vi "Facade.vi"(0 "Data In":T16={"Type"=enum."Tone", "Tone"={"Frequency (kHz)"=0.0, "Phase (cycles)"=0.0, "Random phase"=FALSE}, "Pulse Train"={"Pulse width (us)"=0.0, "Pulse rate (Hz)"=0.0, "Gap (ms)"=0.0, "Polarity"=enum."POS", "PT State"={"Template"=[], "Nperiod"=0, "Index"=0, "Pulse Rate (Hz)"=0.0, "Phase (cycles)"=0.0, "Noff"=0}, "Asynch"=FALSE}, "Noise"={"Properties"={"InvFilt"=FALSE, "Aweight"=FALSE, "Seed"=0, "Tokens"=0, "Brickwall"=FALSE}, "Data"={"TokenNum"=0}}, "File"={"Filename"=path "", "Signal"=[], "Channel"=0, "stream"=FALSE, "offset"=0, "nreps"=0, "loops"=0, "Randomize"=FALSE, "order"=[], "Seed"=0, "Tokens"=0}, "FMSweep"={"Rate (oct/s)"=0.0, "Fmin (Hz)"=0.0, "Fmax (Hz)"=0.0, "Ramp (ms)"=0.0, "Linear"=FALSE}, "Chirp Train"={"Params"={"Fmin (kHz)"=4.0, "Fmax (kHz)"=64.0, "Compensate"=FALSE, "Duration (ms)"=2.0}, "Data"={"WF"=[]}}, "Complex Tone"={"Params"={"F0 (Hz)"=0.0, "Band"={"Flow (Hz)"=0.0, "Fhigh (Hz)"=0.0}, "Phase"=enum."Cosine", "Min F0 (Hz)"=0.0, "Max F0 (Hz)"=0.0, "ContinRandPhase"=FALSE, "Max peak factor"=inf, "Max mod depth"=2.0, "MinHarmNum"=0, "MaxHarmNum"=0, "Level Mode"=enum."per component", "% jitter"=0.0}, "Data"={"Ncomp"=0, "MinHarm"=0, "Phase"=[], "Amplitude"=[], "Npts/frame"=0, "Last F0"=0.0, "Fmin"=0.0, "Fmax"=0.0, "Lslope"=0.0, "randphase"=FALSE, "overall rms"=FALSE, "fmult"=[], "jittered"=FALSE}}, "FM"={"Carrier (kHz)"=0.0, "ModRate (Hz)"=0.0, "Depth (Hz)"=0.0, "Phase (cycles)"=0.0}, "Vowel"={"Freqs"="", "Set level"=enum."Total", "Freq"=[], "weights"=[]}, "Ramp"={"Duration (ms)"=0.0}}, 2 "Display State In":T13, 3 "Container State":T15) -> (6 "Data Out":T16={"Type"=enum."Tone", "Tone"={"Frequency (kHz)"=0.0, "Phase (cycles)"=0.0, "Random phase"=FALSE}, "Pulse Train"={"Pulse width (us)"=0.0, "Pulse rate (Hz)"=0.0, "Gap (ms)"=0.0, "Polarity"=enum."POS", "PT State"={"Template"=[], "Nperiod"=0, "Index"=0, "Pulse Rate (Hz)"=0.0, "Phase (cycles)"=0.0, "Noff"=0}, "Asynch"=FALSE}, "Noise"={"Properties"={"InvFilt"=FALSE, "Aweight"=FALSE, "Seed"=0, "Tokens"=0, "Brickwall"=FALSE}, "Data"={"TokenNum"=0}}, "File"={"Filename"=path "", "Signal"=[], "Channel"=0, "stream"=FALSE, "offset"=0, "nreps"=0, "loops"=0, "Randomize"=FALSE, "order"=[], "Seed"=0, "Tokens"=0}, "FMSweep"={"Rate (oct/s)"=0.0, "Fmin (Hz)"=0.0, "Fmax (Hz)"=0.0, "Ramp (ms)"=0.0, "Linear"=FALSE}, "Chirp Train"={"Params"={"Fmin (kHz)"=4.0, "Fmax (kHz)"=64.0, "Compensate"=FALSE, "Duration (ms)"=2.0}, "Data"={"WF"=[]}}, "Complex Tone"={"Params"={"F0 (Hz)"=0.0, "Band"={"Flow (Hz)"=0.0, "Fhigh (Hz)"=0.0}, "Phase"=enum."Cosine", "Min F0 (Hz)"=0.0, "Max F0 (Hz)"=0.0, "ContinRandPhase"=FALSE, "Max peak factor"=inf, "Max mod depth"=2.0, "MinHarmNum"=0, "MaxHarmNum"=0, "Level Mode"=enum."per component", "% jitter"=0.0}, "Data"={"Ncomp"=0, "MinHarm"=0, "Phase"=[], "Amplitude"=[], "Npts/frame"=0, "Last F0"=0.0, "Fmin"=0.0, "Fmax"=0.0, "Lslope"=0.0, "randphase"=FALSE, "overall rms"=FALSE, "fmult"=[], "jittered"=FALSE}}, "FM"={"Carrier (kHz)"=0.0, "ModRate (Hz)"=0.0, "Depth (Hz)"=0.0, "Phase (cycles)"=0.0}, "Vowel"={"Freqs"="", "Set level"=enum."Total", "Freq"=[], "weights"=[]}, "Ramp"={"Duration (ms)"=0.0}}, 7 "Display State Out":T13, 8 "Action":T12)   [LabVIEW 2020, in "Waveform (G3).xctl"]
uses:
  Waveform (G3).xctl
  Waveform Data.ctl
  Waveform VIs/Waveform Enum (V3).ctl
  Tone (G3)/Tone.Properties.ctl
  Waveform VIs/Pulse Train VIs/Pulse Train Params.ctl
  Waveform VIs/Pulse Train VIs/Pulse Polarity.ctl
  Waveform VIs/Pulse Train VIs/PT-Continuous State.ctl
  Waveform VIs/Noise VIs/Noise (G3).ctl
  Waveform VIs/Noise VIs/Noise (G3).Properties.ctl
  Waveform VIs/Noise VIs/Noise (G3).Data.ctl
  Waveform VIs/File VIs/StimFile-Params.ctl
  Waveform VIs/FM Sweep VIs/FM Sweep Params.ctl
  Waveform VIs/Chirp Train VIs/Chirp Train.ctl
  Waveform VIs/Chirp Train VIs/Chirp Train Params.ctl
  Waveform VIs/Complex Tone VIs/CT-Params.ctl
  Waveform VIs/Complex Tone VIs/CT-Phase Enum.ctl
  Waveform VIs/Complex Tone VIs/CT-Runtime Data.ctl
  FM Tone/Data.ctl
  Vowel/Vowel.Properties.ctl
  Waveform VIs/Ramp VIs/Ramp.Properties.ctl
  <vilib>/_xctls/Container State.ctl
  State.ctl
  Utility VIs/Controls/KRing/KRing.xctl
  Tone (G3)/Tone (G3).xctl
  Noise (G3)/Noise (G3).xctl
  Noise (G3)/Noise (G3) - Persistent.ctl
  <vilib>/_xctls/Action.ctl
  FM Tone/FM Tone.xctl
  Vowel/Vowel.xctl
  <vilib>/_xctls/XControlSupport.lvlib
panel:
  out "display state signal":bool
  in  "Waveform":i16(xcontrol)
  in  "Tab Control":T1(tab)
  in  "Tone (G3)":T2(xcontrol)
  in  "Noise (G3)":T3(xcontrol)
  in  "Pulse Train Params":T4
  in  "File Params":T7
  in  "FMSweep":T8
  in  "Chirp Train Params":T9={"Fmin (kHz)"=4.0, "Fmax (kHz)"=64.0, "Compensate"=FALSE, "Duration (ms)"=2.0}
  in  "FM Tone":T10(xcontrol)
  in  "Vowel":T11(xcontrol)
  in  "Ramp":cluster{"Duration (ms)":dbl}
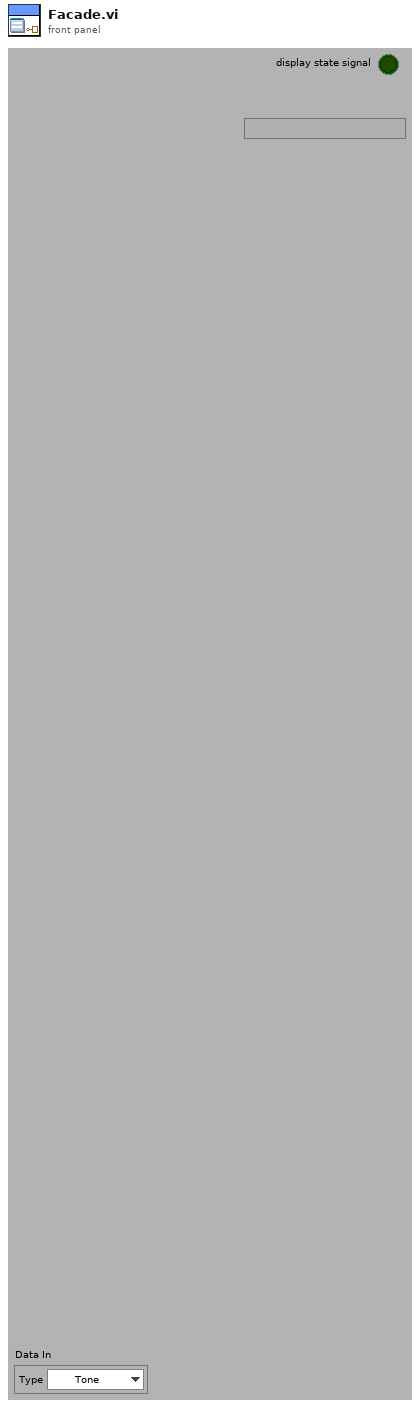
[diagram p1: front panel]
types:
  T1 = enum32{"OFF", "Tone", "Noise", "Pulse train", "File", "FM Sweep", "Chirp", "Complex Tone", "FM Tone", "Vowel", "Ramp"}
  T2 = cluster{"Frequency (kHz)":dbl, "Phase (cycles)":dbl, "Random phase":bool}
  T3 = cluster{"InvFilt":bool, "Aweight":bool, "Seed":i32, "Tokens":i32, "Brickwall":bool}
  T4 = typedef "Pulse Train Params.ctl" = cluster{"Pulse width (us)":dbl, "Pulse rate (Hz)":dbl, "Gap (ms)":dbl, "Polarity":T5, "PT State":T6, "Asynch":bool}
  T5 = typedef "Pulse Polarity.ctl" = enum16{"POS", "NEG", "POS-NEG", "NEG-POS"}
  T6 = typedef "PT-Continuous State.ctl" = cluster{"Template":dbl[], "Nperiod":i32, "Index":i32, "Pulse Rate (Hz)":dbl, "Phase (cycles)":dbl, "Noff":i32}
  T7 = typedef "StimFile-Params.ctl" = cluster{"Filename":path, "Signal":dbl[], "Channel":i32, "stream":bool, "offset":i32, "nreps":i32, "loops":i32, "Randomize":bool, "order":i32[], "Seed":i32, "Tokens":i32}
  T8 = cluster{"Rate (oct/s)":dbl, "Fmin (Hz)":dbl, "Fmax (Hz)":dbl, "Ramp (ms)":dbl, "Linear":bool}
  T9 = cluster{"Fmin (kHz)":dbl, "Fmax (kHz)":dbl, "Compensate":bool, "Duration (ms)":dbl}
  T10 = cluster{"Carrier (kHz)":dbl, "ModRate (Hz)":dbl, "Depth (Hz)":dbl, "Phase (cycles)":dbl}
  T11 = cluster{"Freqs":string, "Set level":enum16{"Total", "Per component"}, "Freq":dbl[], "weights":dbl[]}
  T12 = typedef "XControlSupport.lvlib/Action.ctl" = cluster{"Data Changed?":bool, "State Changed?":bool, "Action Name":string}
  T13 = typedef "Waveform (G3).xctl/State.ctl" = cluster{"Waveform names":string[], "Valid":bool[], "enable menu":bool, "Controls":cluster{"Type ":refnum<vi>, "Tone ":refnum<vi>, "Noise":refnum<vi>}, "persistent":cluster{"noise":T14, "Sort":bool}, "multi":bool}
  T14 = typedef "Noise (G3).xctl/Noise (G3) - Persistent.ctl" = cluster{"Show Aweight":bool}
  T15 = typedef "XControlSupport.lvlib/Container State.ctl" = cluster{"Indicator?":bool, "Run Mode?":bool, " Refnum":refnum<vi>}
  T16 = typedef "Waveform (G3).xctl/Waveform Data.ctl" = cluster{"Type":T17, "Tone":T18, "Pulse Train":T4, "Noise":T19, "File":T7, "FMSweep":T22, "Chirp Train":T23, "Complex Tone":cluster{"Params":T25, "Data":T27}, "FM":T28, "Vowel":T29, "Ramp":T30}
  T17 = typedef "Waveform Enum (V3).ctl" = enum16{"OFF", "Tone", "Noise", "Pulse Train", "File", "FM Sweep", "Chirp Train", "Complex Tone", "FM Tone", "Vowel", "Ramp"}
  T18 = typedef "Tone (G3).xctl/Tone.Properties.ctl" = cluster{"Frequency (kHz)":dbl, "Phase (cycles)":dbl, "Random phase":bool}
  T19 = typedef "Noise (G3).ctl" = cluster{"Properties":T20, "Data":T21}
  T20 = typedef "Noise (G3).Properties.ctl" = cluster{"InvFilt":bool, "Aweight":bool, "Seed":i32, "Tokens":i32, "Brickwall":bool}
  T21 = typedef "Noise (G3).Data.ctl" = cluster{"TokenNum":i32}
  T22 = typedef "FM Sweep Params.ctl" = cluster{"Rate (oct/s)":dbl, "Fmin (Hz)":dbl, "Fmax (Hz)":dbl, "Ramp (ms)":dbl, "Linear":bool}
  T23 = typedef "Chirp Train.ctl" = cluster{"Params":T24, "Data":cluster{"WF":dbl[]}}
  T24 = typedef "Chirp Train Params.ctl" = cluster{"Fmin (kHz)":dbl, "Fmax (kHz)":dbl, "Compensate":bool, "Duration (ms)":dbl}
  T25 = typedef "CT-Params.ctl" = cluster{"F0 (Hz)":dbl, "Band":cluster{"Flow (Hz)":dbl, "Fhigh (Hz)":dbl}, "Phase":T26, "Min F0 (Hz)":dbl, "Max F0 (Hz)":dbl, "ContinRandPhase":bool, "Max peak factor":dbl, "Max mod depth":dbl, "MinHarmNum":i32, "MaxHarmNum":i32, "Level Mode":enum16{"per component", "overall rms"}, "% jitter":dbl}
  T26 = typedef "CT-Phase Enum.ctl" = enum16{"Cosine", "Random", "Alternating"}
  T27 = typedef "CT-Runtime Data.ctl" = cluster{"Ncomp":i32, "MinHarm":i32, "Phase":dbl[], "Amplitude":dbl[], "Npts/frame":i32, "Last F0":dbl, "Fmin":dbl, "Fmax":dbl, "Lslope":dbl, "randphase":bool, "overall rms":bool, "fmult":dbl[], "jittered":bool}
  T28 = typedef "FM Tone.xctl/Data.ctl" = cluster{"Carrier (kHz)":dbl, "ModRate (Hz)":dbl, "Depth (Hz)":dbl, "Phase (cycles)":dbl}
  T29 = typedef "Vowel.xctl/Vowel.Properties.ctl" = cluster{"Freqs":string, "Set level":enum16{"Total", "Per component"}, "Freq":dbl[], "weights":dbl[]}
  T30 = typedef "Ramp.Properties.ctl" = cluster{"Duration (ms)":dbl}
  T31 = enum32{"OFF", "Tone", "Noise", "Pulse train", "File", "FM Sweep", "Chirp", "Complex Tone", "FM Tone"}
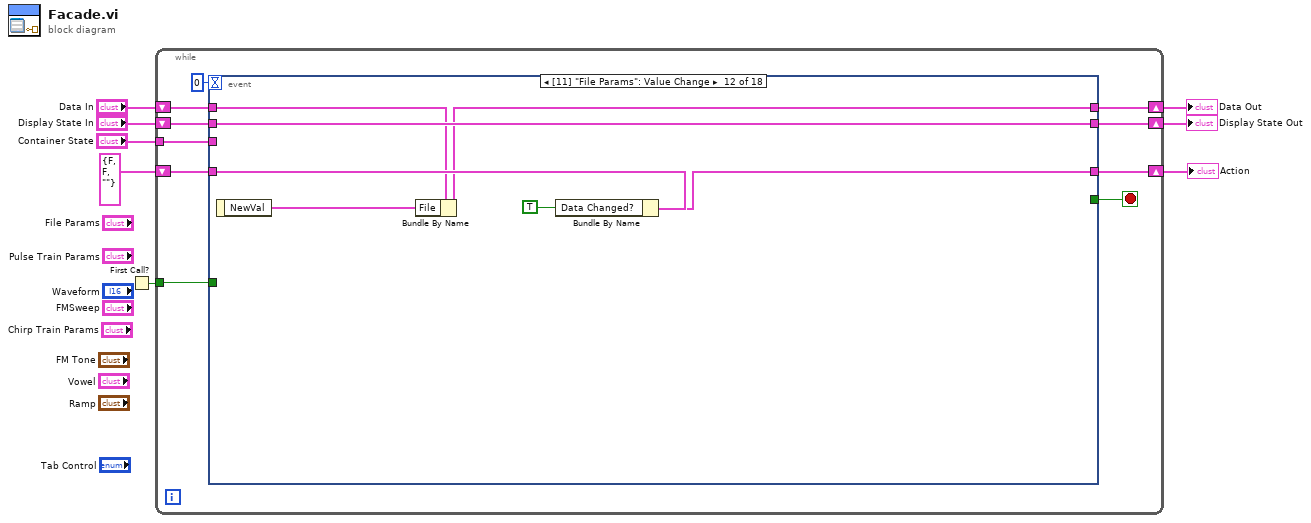
[diagram p0: block diagram]
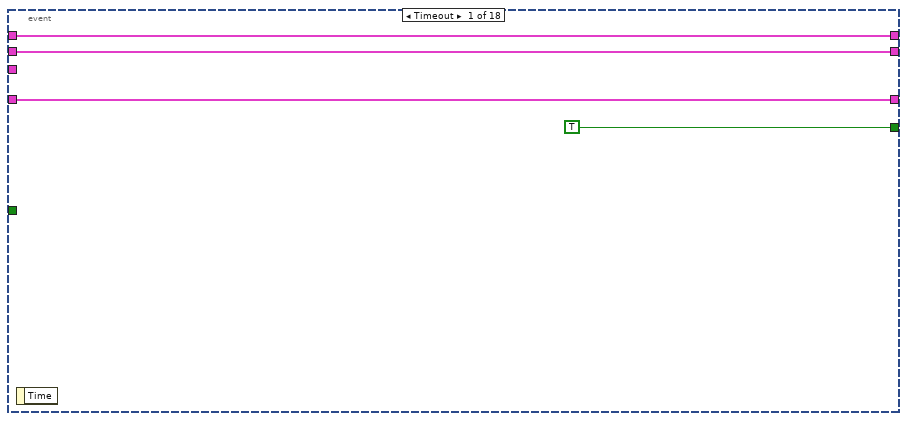
[diagram p2: hidden frame]
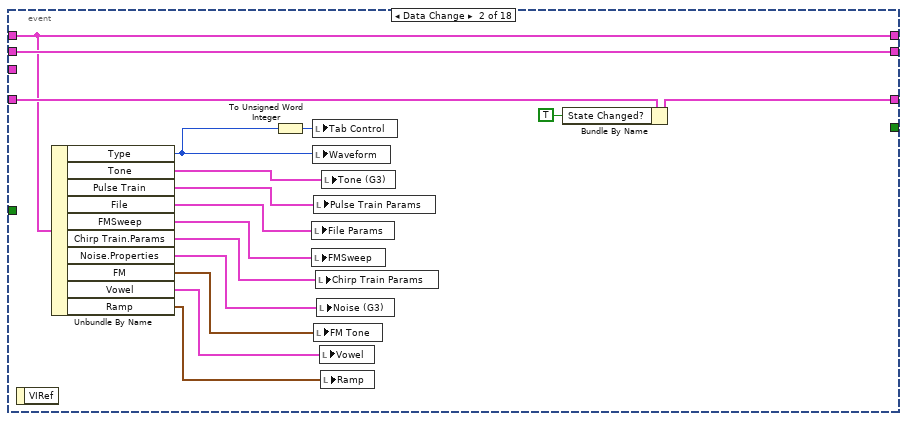
[diagram p3: hidden frame]
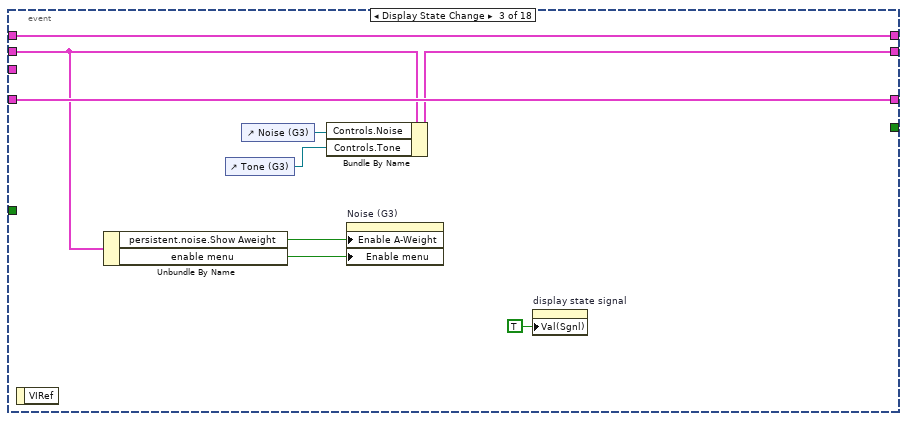
[diagram p4: hidden frame]
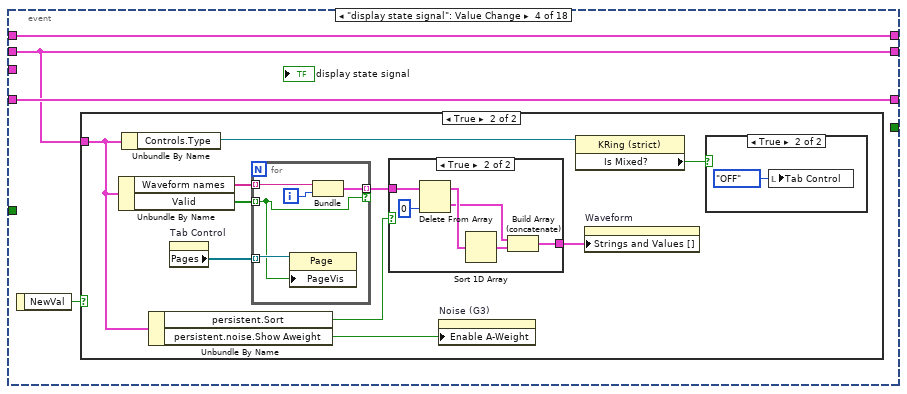
[diagram p5: hidden frame]
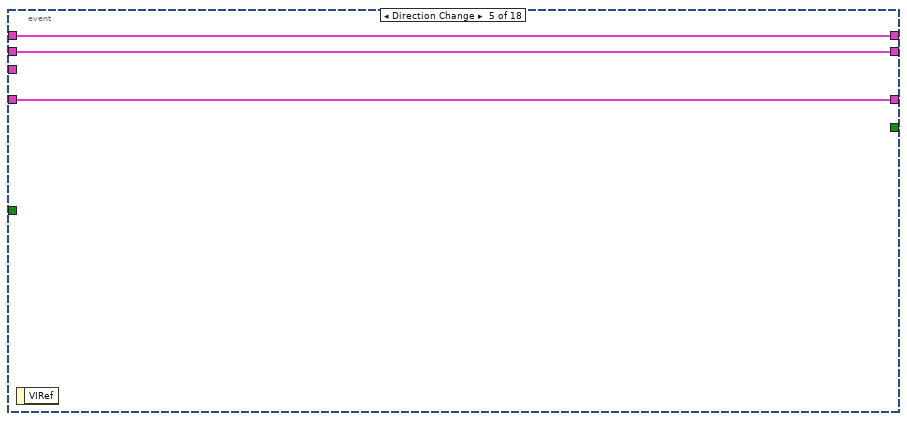
[diagram p9: hidden frame]
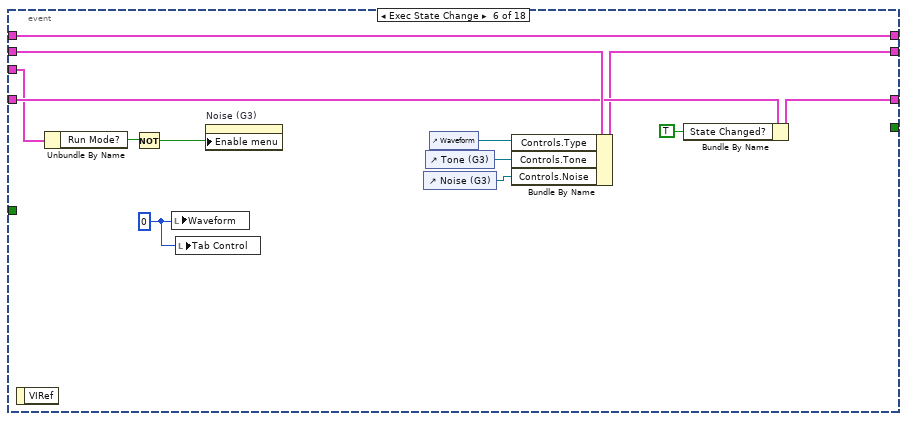
[diagram p10: hidden frame]
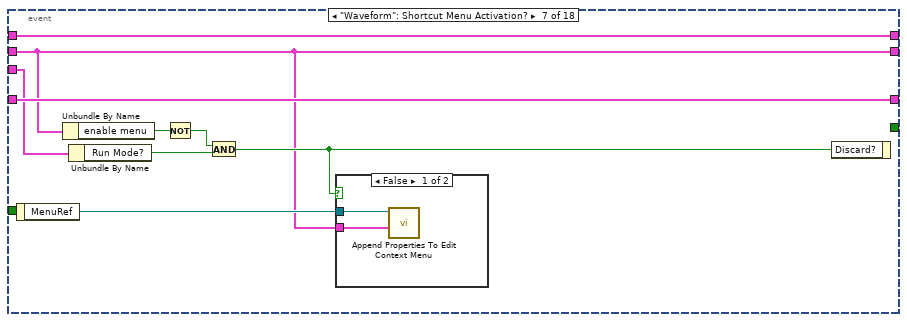
[diagram p11: hidden frame]
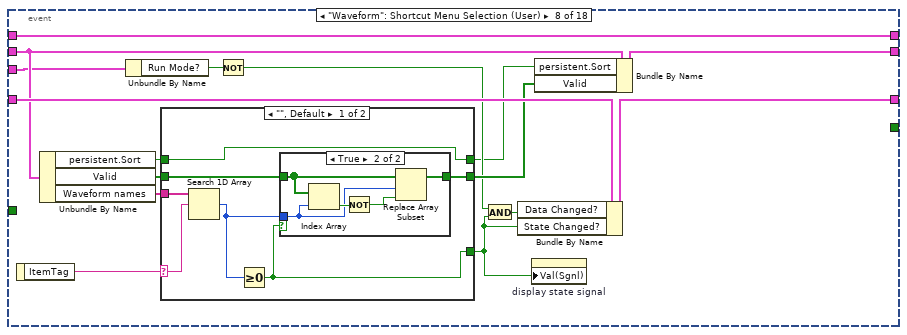
[diagram p13: hidden frame]
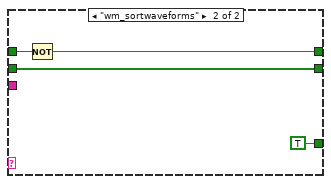
[diagram p15: hidden frame]
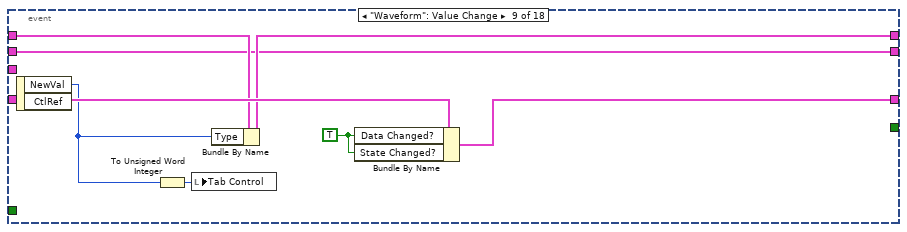
[diagram p16: hidden frame]
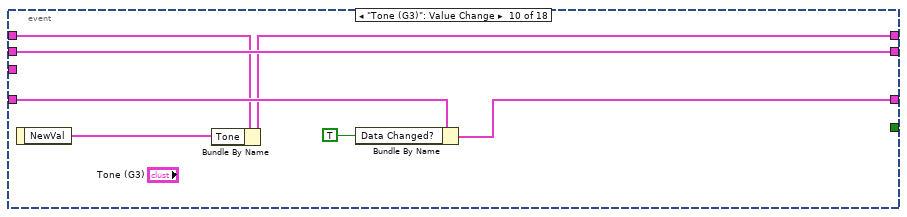
[diagram p17: hidden frame]
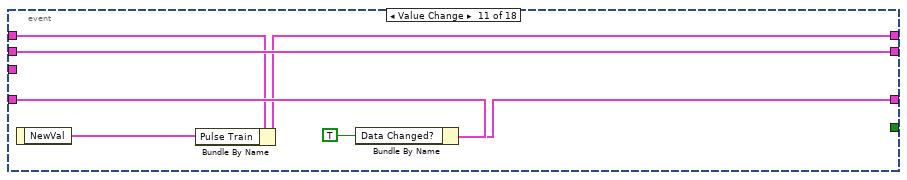
[diagram p18: hidden frame]
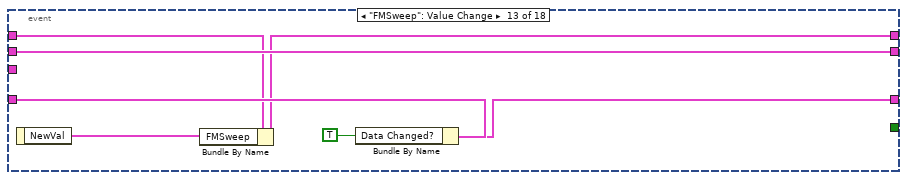
[diagram p19: hidden frame]
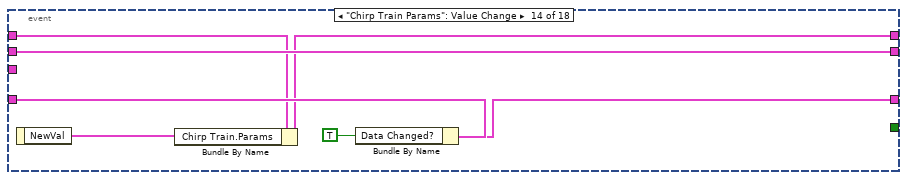
[diagram p20: hidden frame]
diagram:
  n1 = First Call?() -> (First Call?: T/F=w1:bool)
  n2 = while {
    shift-right: [w17] -> w5
    shift-left: "Display State In" -> [w18]
    tunnel: "Container State" -> [w14]
    shift-right: [w12] -> w8
    shift-left: "Data In" -> [w13]
    shift-right: [w10] -> w3
    shift-left: T12 {"Data Changed?"=FALSE, "State Changed?"=FALSE, "Action Name"=""} ("Action") -> [w11]
    tunnel: w1 -> [w9]
    stop <- w16 stop-if-true
    n3 = event shown="[11] \"File Params\": Value Change" {
      selector: _ -> [_ _ _ _ _ _ _ _ _ _ _ _ _ _ _ _ _ _]
      dyn-events: _ -> [_ _ _ _ _ _ _ _ _ _ _ _ _ _ _ _ _ _]
      timeout: 0 -> [_ _ _ _ _ _ _ _ _ _ _ _ _ _ _ _ _ _]
      tunnel: w18 -> [w20 w38 w42 w48 w77 w90 w94 w111 w137 w149 w156 w163 w170 w177 w185 w193 w200 w207]
      tunnel: [w20 w38 w45 w48 w77 w84 w94 w110 w137 w149 w156 w163 w170 w177 w180 w193 w200 w207] -> w17
      tunnel: [TRUE _ _ _ _ _ _ _ _ _ _ _ _ _ _ _ _ _] -> w16
      tunnel: w14 -> [_ _ _ _ _ w87 w97 w108 _ _ _ _ _ _ _ _ _ _]
      tunnel: w13 -> [w19 w36 w47 w51 w76 w89 w99 w117 w140 w145 w152 w159 w166 w173 w186 w192 w199 w206]
      tunnel: [w19 w36 w47 w51 w76 w89 w99 w117 w139 w144 w151 w158 w165 w172 w183 w190 w197 w204] -> w12
      tunnel: [w21 w27 w46 w50 w75 w83 w98 w115 w141 w146 w153 w160 w167 w174 w184 w188 w195 w202] -> w10
      tunnel: w11 -> [w21 w37 w46 w50 w75 w88 w98 w116 w142 w148 w155 w162 w169 w176 w179 w191 w198 w205]
      tunnel: w9 -> [_ _ _ _ _ _ _ _ _ _ _ _ _ _ _ _ _ _]
      event Timeout {
        n4 = event-data() -> ()  [unwired: 1 in, 1 out]
      }
      event Data Change {
        n5 = event-data() -> ()  [unwired: 1 in, 1 out]
        n6 = Unbundle By Name(w36) -> ("Type"=w25:T17, "Tone"=w35:T18, "Pulse Train"=w34:T4, "File"=w32:T7, "FMSweep"=w31:T22, "Chirp Train.Params"=w30:T24, "Noise.Properties"=w29:T20, "FM"=w28:T28, "Vowel"=w24:T29, "Ramp"=w23:T30)
        n7 = To Unsigned Word Integer(number=w25) -> (unsigned 16bit integer=w33:u16)
        n8 = local write "File Params"(w32) -> ()
        n9 = local write "FMSweep"(w31) -> ()
        n10 = local write "Tab Control"(w33) -> ()
        n11 = local write "Waveform"(w25) -> ()
        n12 = local write "Pulse Train Params"(w34) -> ()
        n13 = local write "FM Tone"(w28) -> ()
        n14 = local write "Chirp Train Params"(w30) -> ()
        n15 = local write "Noise (G3)"(w29) -> ()
        n16 = local write "Vowel"(w24) -> ()
        n17 = local write "Ramp"(w23) -> ()
        n18 = local write "Tone (G3)"(w35) -> ()
        n19 = Bundle By Name(cluster=w37, "State Changed?"=TRUE) -> (w27:T12)
      }
      event Display State Change {
        n20 = event-data() -> ()  [unwired: 1 in, 1 out]
        n21 = Unbundle By Name(w42) -> ("persistent.noise.Show Aweight"=w41:bool, "enable menu"=w40:bool)
        n22 = control-ref of="Tone (G3)"() -> (w39:refnum<vi>)
        n23 = control-ref of="Noise (G3)"() -> (w44:refnum<vi>)
        n24 = Bundle By Name(cluster=w42, "Controls.Noise"=w44, "Controls.Tone"=w39) -> (w45:T13)
        n25 = property on="Noise (G3)" class="Noise (G3) (strict)"("Enable A-Weight"=w41, "Enable menu"=w40) -> ()  [unwired: 2 in, 2 out]
        n26 = property on="display state signal" class="Bool (strict)"("Val(Sgnl)"=TRUE ("Value (Signaling)")) -> ()  [unwired: 2 in, 2 out]
      }
      event "display state signal": Value Change {
        n27 = event-data() -> ("NewVal"=w49:bool)  [unwired: 1 in]
        n28 = case shown="True" w49 {
          tunnel: w48 -> [_ w55]
          frame False {
          }
          frame True {
            n29 = Unbundle By Name(w55) -> ("Waveform names"=w60:string[], "Valid"=w61:bool[])
            n30 = Unbundle By Name(w55) -> ("Controls.Type"=w53:refnum<vi>)
            n31 = Unbundle By Name(w55) -> ("persistent.Sort"=w56:bool, "persistent.noise.Show Aweight"=w58:bool)
            n32 = property on="Tab Control" class="TabCtl (strict)"() -> ("Pages"=w59:refnum<vi>[])  [unwired: 2 in, 2 out]
            n33 = for {
              tunnel: w61 -> [w70] mode=indexing
              tunnel: w60 -> [w71] mode=indexing
              tunnel: [w74] -> w57 mode=indexing if=w70
              tunnel: w59 -> [w72] mode=indexing
              i -> [w73]
              n34 = property class="Page"(reference=w72, "PageVis"=w70) -> ()  [unwired: 1 in, 2 out]
              n35 = Bundle("String"=w71, w73) -> (w74:cluster{"String":string, i32})  [unwired: 1 in]
            }
            n36 = case shown="True" w56 {
              tunnel: w57 -> [w63 w69]
              tunnel: [w63 w64] -> w54
              frame False {
              }
              frame True {
                n37 = Delete From Array(array=w69, index=0) -> (deleted portion=w65:cluster{"String":string, i32}, array with subset deleted=w67:cluster{"String":string, i32}[])  [unwired: 1 in]
                n38 = Sort 1D Array(array=w67) -> (sorted array=w66:cluster{"String":string, i32}[])
                n39 = Build Array (concatenate)(w65, w66) -> (w64:cluster{"String":string, i32}[])
              }
            }
            n40 = property on="Noise (G3)" class="Noise (G3) (strict)"("Enable A-Weight"=w58) -> ()  [unwired: 2 in, 2 out]
            n41 = property class="KRing (strict)"(reference=w53) -> ("Is Mixed?"=w52:bool)  [unwired: 1 in, 2 out]
            n42 = property on="Waveform" class="KRing (strict)"("Strings and Values []"=w54) -> ()  [unwired: 2 in, 2 out]
            n43 = case shown="True" w52 {
              frame False {
              }
              frame True {
                n44 = local write "Tab Control"(T31."OFF" ("Tab Control")) -> ()
              }
            }
          }
        }
      }
      event Direction Change {
        n45 = event-data() -> ()  [unwired: 1 in, 1 out]
      }
      event Exec State Change {
        w81 = 0
        n46 = event-data() -> ()  [unwired: 1 in, 1 out]
        n47 = Unbundle By Name(w87) -> ("Run Mode?"=w86:bool)
        n48 = Not(x=w86) -> (.not. x?=w85:bool)
        n49 = local write "Waveform"(w81) -> ()
        n50 = local write "Tab Control"(w81) -> ()
        n51 = property on="Noise (G3)" class="Noise (G3) (strict)"("Enable menu"=w85) -> ()  [unwired: 2 in, 2 out]
        n52 = control-ref of="Noise (G3)"() -> (w78:refnum<vi>)
        n53 = control-ref of="Tone (G3)"() -> (w80:refnum<vi>)
        n54 = control-ref of="Waveform"() -> (w79:refnum<vi>)
        n55 = Bundle By Name(cluster=w90, "Controls.Type"=w79, "Controls.Tone"=w80, "Controls.Noise"=w78) -> (w84:T13)
        n56 = Bundle By Name(cluster=w88, "State Changed?"=TRUE) -> (w83:T12)
      }
      event "Waveform": Shortcut Menu Activation? {
        n57 = event-data() -> ("MenuRef"=w96:refnum<k9>)  [unwired: 1 in]
        n58 = Unbundle By Name(w94) -> ("enable menu"=w92:bool)
        n59 = Unbundle By Name(w97) -> ("Run Mode?"=w93:bool)
        n60 = Not(x=w92) -> (.not. x?=w91:bool)
        n61 = And(x=w91, y=w93) -> (x .and. y?=w95:bool)
        n62 = case shown="False" w95 {
          tunnel: w94 -> [w100 _]
          tunnel: w96 -> [w101 _]
          frame False {
            n63 = call "Append Properties To Edit Context Menu.vi"("State"=w100, "Menu in"=w101) -> ()  [unwired: 10 in]
          }
          frame True {
          }
        }
        n64 = event-data("Discard?"=w95) -> ()  [unwired: 1 in, 1 out]
      }
      event "Waveform": Shortcut Menu Selection (User) {
        n65 = event-data() -> ("ItemTag"=w113:string)  [unwired: 1 in]
        n66 = Unbundle By Name(w111) -> ("persistent.Sort"=w103:bool, "Valid"=w112:bool[], "Waveform names"=w114:string[])
        n67 = Unbundle By Name(w108) -> ("Run Mode?"=w106:bool)
        n68 = case shown="\"\", Default" w113 {
          selector: w113 -> [w123 _]
          tunnel: w114 -> [w124 _]
          tunnel: w112 -> [w122 w134]
          tunnel: [w120 w134] -> w109
          tunnel: [w119 TRUE] -> w104
          tunnel: w103 -> [w118 w132]
          tunnel: [w118 w131] -> w102
          frame "", Default {
            n69 = Search 1D Array(1D array=w124, element=w123) -> (index of element=w121:i32)  [unwired: 1 in]
            n70 = Greater Or Equal To 0?(x=w121) -> (x >= 0?=w119:bool)
            n71 = case shown="True" w119 {
              tunnel: w122 -> [w125 w128]
              tunnel: w121 -> [_ w126]
              tunnel: [w125 w127] -> w120
              frame False {
              }
              frame True {
                n72 = Index Array(array=w128, index=w126) -> (element=w130:bool)
                n73 = Not(x=w130) -> (.not. x?=w129:bool)
                n74 = Replace Array Subset(array=w128, new element=w129, index=w126) -> (w127:bool[])
              }
            }
          }
          frame "wm_sortwaveforms" {
            n75 = Not(x=w132) -> (.not. x?=w131:bool)
          }
        }
        n76 = Not(x=w106) -> (.not. x?=w105:bool)
        n77 = And(x=w105, y=w104) -> (x .and. y?=w107:bool)
        n78 = Bundle By Name(cluster=w116, "Data Changed?"=w107, "State Changed?"=w104) -> (w115:T12)
        n79 = property on="display state signal" class="Bool (strict)"("Val(Sgnl)"=w104) -> ()  [unwired: 2 in, 2 out]
        n80 = Bundle By Name(cluster=w111, "persistent.Sort"=w102, "Valid"=w109) -> (w110:T13)
      }
      event "Waveform": Value Change {
        w135 = TRUE ("Data Changed?")
        n81 = event-data() -> ("NewVal"=w136:i16)  [unwired: 1 in, 1 out]
        n82 = To Unsigned Word Integer(number=w136) -> (unsigned 16bit integer=w138:u16)
        n83 = local write "Tab Control"(w138) -> ()
        n84 = Bundle By Name(cluster=w140, "Type"=w136) -> (w139:T16)
        n85 = Bundle By Name(cluster=w142, "Data Changed?"=w135, "State Changed?"=w135) -> (w141:T12)
      }
      event "Tone (G3)": Value Change {
        n86 = event-data() -> ("NewVal"=w143:T2)  [unwired: 1 in]
        n87 = Bundle By Name(cluster=w145, "Tone"=w143) -> (w144:T16)
        n88 = Bundle By Name(cluster=w148, "Data Changed?"=TRUE) -> (w146:T12)
      }
      event Value Change {
        n89 = event-data() -> ("NewVal"=w150:T4)  [unwired: 1 in]
        n90 = Bundle By Name(cluster=w152, "Pulse Train"=w150) -> (w151:T16)
        n91 = Bundle By Name(cluster=w155, "Data Changed?"=TRUE) -> (w153:T12)
      }
      event Value Change {
        n92 = event-data() -> ("NewVal"=w157:T7)  [unwired: 1 in]
        n93 = Bundle By Name(cluster=w159, "File"=w157) -> (w158:T16)
        n94 = Bundle By Name(cluster=w162, "Data Changed?"=TRUE) -> (w160:T12)
      }
      event "FMSweep": Value Change {
        n95 = event-data() -> ("NewVal"=w164:T8)  [unwired: 1 in]
        n96 = Bundle By Name(cluster=w166, "FMSweep"=w164) -> (w165:T16)
        n97 = Bundle By Name(cluster=w169, "Data Changed?"=TRUE) -> (w167:T12)
      }
      event "Chirp Train Params": Value Change {
        n98 = event-data() -> ("NewVal"=w171:T9)  [unwired: 1 in]
        n99 = Bundle By Name(cluster=w173, "Chirp Train.Params"=w171) -> (w172:T16)
        n100 = Bundle By Name(cluster=w176, "Data Changed?"=TRUE) -> (w174:T12)
      }
      event "Noise (G3)": Value Change {
        w181 = TRUE ("Data Changed?")
        n101 = event-data() -> ()  [unwired: 1 in, 1 out]
        n102 = Bundle By Name(cluster=w186, "Noise.Properties"="Noise (G3)") -> (w183:T16)
        n103 = property on="Noise (G3)" class="Noise (G3) (strict)"() -> ("Enable A-Weight"=w178:bool)  [unwired: 2 in, 2 out]
        n104 = Bundle By Name(cluster=w185, "persistent.noise.Show Aweight"=w178) -> (w180:T13)
        n105 = Bundle By Name(cluster=w179, "Data Changed?"=w181, "State Changed?"=w181) -> (w184:T12)
      }
      event "FM Tone": Value Change {
        n106 = event-data() -> ("NewVal"=w189:T10)  [unwired: 1 in]
        n107 = Bundle By Name(cluster=w191, "Data Changed?"=TRUE) -> (w188:T12)
        n108 = Bundle By Name(cluster=w192, "FM"=w189) -> (w190:T16)
      }
      event "Vowel": Value Change {
        n109 = event-data() -> ("NewVal"=w196:T11)  [unwired: 1 in]
        n110 = Bundle By Name(cluster=w198, "Data Changed?"=TRUE) -> (w195:T12)
        n111 = Bundle By Name(cluster=w199, "Vowel"=w196) -> (w197:T16)
      }
      event "Ramp": Value Change {
        n112 = event-data() -> ("NewVal"=w203:cluster{"Duration (ms)":dbl})  [unwired: 1 in]
        n113 = Bundle By Name(cluster=w205, "Data Changed?"=TRUE) -> (w202:T12)
        n114 = Bundle By Name(cluster=w206, "Ramp"=w203) -> (w204:T16)
      }
    }
  }
  "Display State Out" <- w5
  "Data Out" <- w8
  "Action" <- w3
